vi "Archive Filename.vi"(8 "error in (no error)":errorcluster) -> (0 "error out":errorcluster, 3 "filename":string)   [LabVIEW 2013]
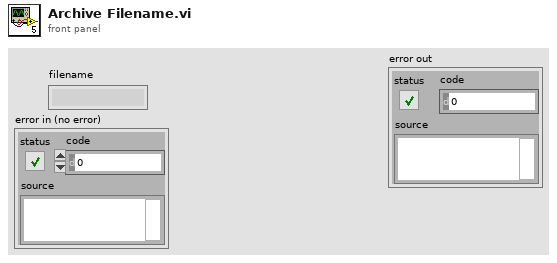
[diagram p1: front panel]
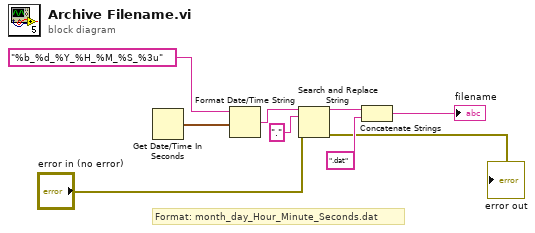
[diagram p0: block diagram]
diagram:
  # "Format: month_day_Hour_Minute_Seconds.dat"
  n1 = Get Date/Time In Seconds() -> (seconds since 1Jan1904=w9:timestamp)
  n2 = Format Date/Time String(time format string (%c)="%b_%d_%Y_%H_%M_%S_%3u", seconds (now)=w9) -> (date/time string=w7:string)  [unwired: 1 in]
  n3 = Search and Replace String(input string=w7, search string=".", error in="error in (no error)") -> (result string=w5:string, error out=→"error out":errorcluster)  [unwired: 5 in, 2 out]
  n4 = Concatenate Strings(w5, ".dat" ("string")) -> (→"filename":string)
